vi "CanGrabberSetpoint.vi"() -> ()   [LabVIEW 2014]
panel:
  in  "Can Gabber Setpoint":dbl
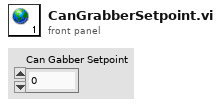
[diagram p1: front panel]
diagram:
